vi "UART Check Number of Ports.vi"(0 "UART Driver in":refnum<class "UART Driver.lvclass">, 11 "error in":errorcluster) -> (4 "UART Driver out":refnum<class "UART Driver.lvclass">, 15 "error out":errorcluster)   [LabVIEW 2012, in "UART_Host_Driver.lvlib" / "UART Driver.lvclass"]
doc: "Check the Number of Ports against what the Number of Ports supported by the FPGA personality."
uses:
  UART Driver.lvclass
  Typedefs/FPGA VI Reference.ctl
  UART Driver.lvclass/UART Driver.ctl
  <vilib>/Utility/error.llb/Error Cluster From Error Code.vi
  <vilib>/rvi/errors/niLvFpgaAdjustHostInterfaceError.vi
  <vilib>/rvi/interface/nirviReadWriteControl/nirviReadWriteControl.xnode
  <vilib>/ErrorRing/Error Ring.xnode
  UART_Host_Driver.lvlib
  NiFpgaLv.dll
  <vilib>/rvi/interface/Simulation/niFpgaSimulationCallBeginRW.vi
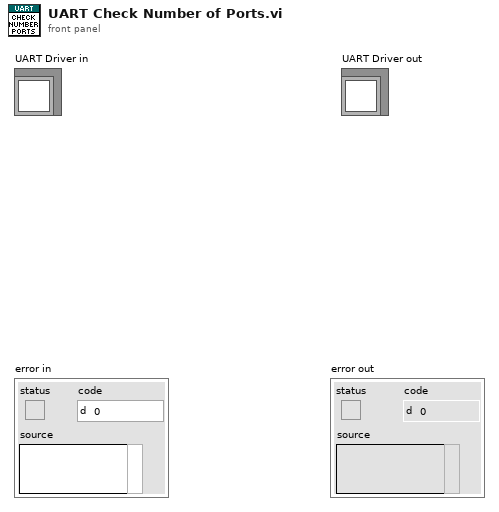
[diagram p1: front panel]
types:
  T1 = typedef "UART_Host_Driver.lvlib/FPGA VI Reference.ctl" = refnum<k20>
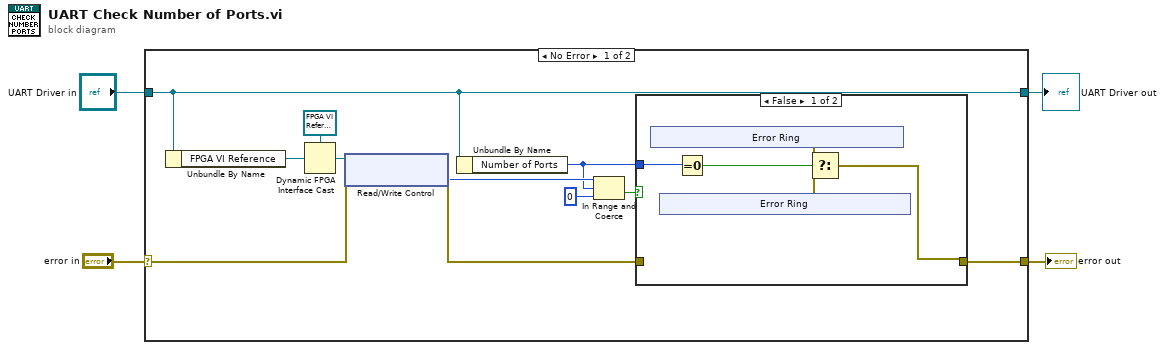
[diagram p0: block diagram]
diagram:
  n1 = case shown="No Error" "error in" {
    selector: "error in" -> [w12 w31]
    tunnel: [w9 w31] -> w3
    tunnel: [w11 w30] -> w2
    tunnel: "UART Driver in" -> [w11 w30]
    frame No Error {
      n2 = Unbundle By Name(w11) -> ("FPGA VI Reference"=w15:refnum<k20>)
      n3 = Dynamic FPGA Interface Cast(Session In=T1 refnum ("FPGA VI Reference"), Type=w15) -> (Session Out=w13:T1)
      n4 = xnode "Read/Write Control"("FPGA VI Reference In"=w13, "error in"=w12) -> ("error out"=w10:errorcluster, "Maximum Nup?"=w8:u8)  [unwired: 1 out]
      n5 = Unbundle By Name(w11) -> ("Number of Ports"=w5:u8)
      n6 = In Range and Coerce(upper limit=w8, x=w5, lower limit=u8 0) -> (In Range?=w6:bool)  [unwired: 1 out]
      n7 = case shown="False" w6 {
        tunnel: w10 -> [_ w29]
        tunnel: [w17 w29] -> w9
        tunnel: w5 -> [w20 _]
        frame False {
          n8 = xnode "Error Ring"() -> ("error out"=w16:errorcluster)
          n9 = xnode "Error Ring"() -> ("error out"=w18:errorcluster)
          n10 = Equal To 0?(x=w20) -> (x = 0?=w19:bool)
          n11 = Select(t=w16, s=w19, f=w18) -> (s? t:f=w17:errorcluster)
        }
        frame True {
        }
      }
    }
    frame Error {
    }
  }
  "error out" <- w3
  "UART Driver out" <- w2
